vi "ASCII_To_Hex(NUM).vi"(11 "ASCII NUM":u8) -> (3 "hex1":u8)   [LabVIEW 2013]
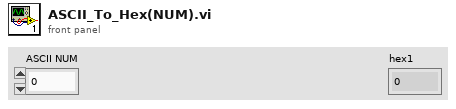
[diagram p1: front panel]
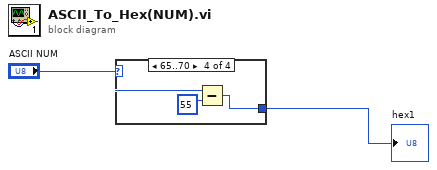
[diagram p0: block diagram]
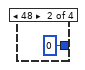
[diagram p3: hidden frame]
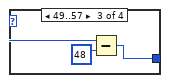
[diagram p4: hidden frame]
diagram:
  n1 = case shown="65..70" "ASCII NUM" {
    selector: "ASCII NUM" -> [w3 _ w7 w10]
    tunnel: [w3 u8 0 w5 w8] -> w2
    frame 0, Default {
    }
    frame 48 {
    }
    frame 49..57 {
      n2 = Subtract(x=w7, y=u8 48) -> (x-y=w5:u8)
    }
    frame 65..70 {
      n3 = Subtract(x=w10, y=u8 55) -> (x-y=w8:u8)
    }
  }
  "hex1" <- w2
